vi "Should Continue.vi"(8 "error in (no error)":errorcluster, 11 "ContinuousDirector in":refnum<class "ContinuousDirector.lvclass">) -> (0 "error out":errorcluster, 2 "Should Continue":bool=TRUE, 3 "ContinuousDirector out":refnum<class "ContinuousDirector.lvclass">)   [LabVIEW 2023, in "HAF.lvlib" / "ContinuousDirector.lvclass"]
doc: "Returns true as this Director will continually process Commands."
uses:
  ContinuousDirector.lvclass
  ContinuousDirector.lvclass/ContinuousDirector.ctl
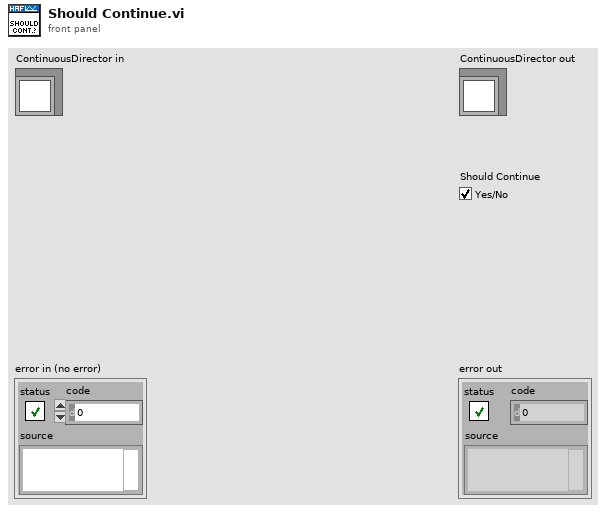
[diagram p1: front panel]
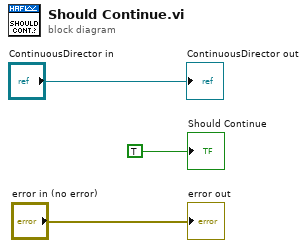
[diagram p0: block diagram]
diagram:
  "error out" <- "error in (no error)"
  "ContinuousDirector out" <- "ContinuousDirector in"
  "Should Continue" <- TRUE ("Should Continue")
